vi "Receive Message.vi"(6 "priority":i32, 10 "Topic in":refnum<class "Topic.lvclass">, 11 "Message in":refnum<class "Message.lvclass">) -> (0 "error out":errorcluster, 2 "Actor out":refnum<class "Actor.lvclass">)   [LabVIEW 2017, in "Mediator.lvlib" / "Topic.lvclass"]
doc: "This VI should be overriden ONLY if you are creating a proxy actor for remote transmission. If you are, override this VI to transmit the received message to a new destination, maintaining the given priority."
uses:
  Topic.lvclass
  <vilib>/ActorFramework/Message/Message.lvclass
  <vilib>/ActorFramework/Actor/Actor.lvclass
  Topic Messages/Notify Subscribers Msg/Notify Subscribers Msg.lvclass
  gpm_packages/@cs/event-logger/Source/Composed Log/Types/Log Level.ctl
  gpm_packages/@cs/event-logger/Source/Composed Log/Composed Log.lvlib
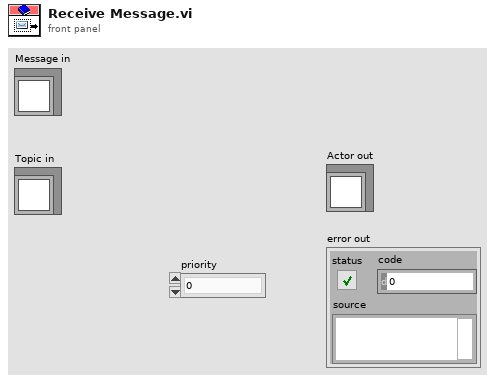
[diagram p1: front panel]
types:
  T1 = typedef "Composed Log.lvlib/Log Level.ctl" = enum16{"Debug", "Info", "Warning", "Error", "Critical"}
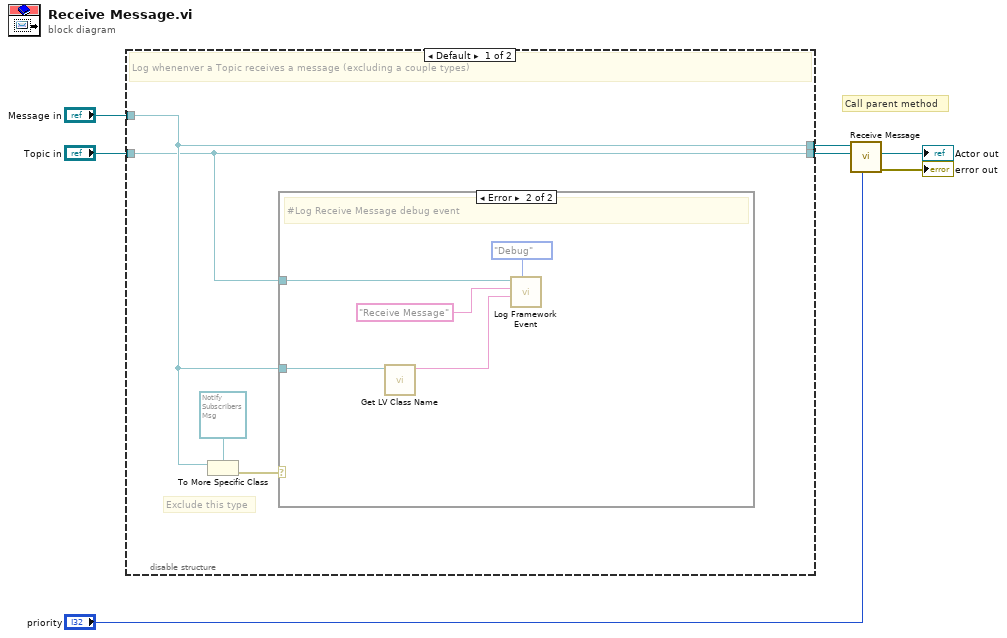
[diagram p0: block diagram]
diagram:
  # "Call parent method"
  n1 = disable-structure shown="Default" {
    disable-tunnel: "Message in" -> [w11 w18]
    disable-tunnel: "Topic in" -> [w8 w17]
    disable-tunnel: [w11 w18] -> w2
    disable-tunnel: [w8 w17] -> w1
    frame condition #0 {
      # "Exclude this type"
      # "Log whenenver a Topic receives a message (excluding a couple types)"
      n2 = To More Specific Class(target class=refnum<class "Notify Subscribers Msg.lvclass"> refnum ("Mediator.lvlib:Notify Subscribers Msg.lvclass"), reference=w11) -> (error out=w9:errorcluster)  [unwired: 1 in, 1 out]
      n3 = case shown="Error" w9 {
        tunnel: w11 -> [_ w12]
        tunnel: w8 -> [_ w13]
        frame No Error {
          # "Exclude logging for mediated datum updates\nbecause there. are. just. too. many. of. them."
          # "Message is a Notify Subscribers Msg -- Do not log this message type"
        }
        frame Error {
          # "#Log Receive Message debug event"
          n4 = call <vilib>:"Get LV Class Name.vi"("object"=w12) -> ("class name"=w14:string)  [unwired: 9 in, 1 out]
          n5 = call "Log Framework Event.vi"("Event Level (Debug)"=Log_Level."Debug", "Data To Log"=w14, "Caller Info (\"\")"="Receive Message" ("Caller Info (\"\")"), "Topic In"=w13) -> ()  [unwired: 7 in, 1 out]
        }
      }
    }
    frame condition #1 (active) {
      # "Remove all logging from this method at compile time"
    }
  }
  n6 = call-parent "Receive Message.vi"("priority"="priority", "Actor in"=w1, "Message in"=w2) -> ("error out"=→"error out":errorcluster, "Actor out"=→"Actor out":refnum<class "Actor.lvclass">)  [unwired: 7 in]
